vi "ddsRControl.vi"(7 "Pre 3.0 AOM driver version?":bool, 8 "Register":dbl min=0.0 max=16.0 step=1.0 format="%#.1f", 9 "DDS: ProgramChanges":bool, 10 "Lock Amp":bool, 11 "Table/Sequence":bool) -> (0 "Software Trigger":string, 3 "Characters for FPGA":string="L00\r\n")   [LabVIEW 2013, in "DDS9954_v2013.lvlib"]
uses:
  DDS9954_v2013.lvlib
  dataToAscii_8bit.vi
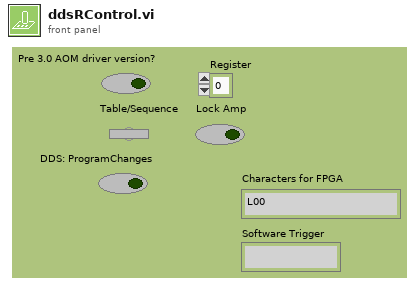
[diagram p1: front panel]
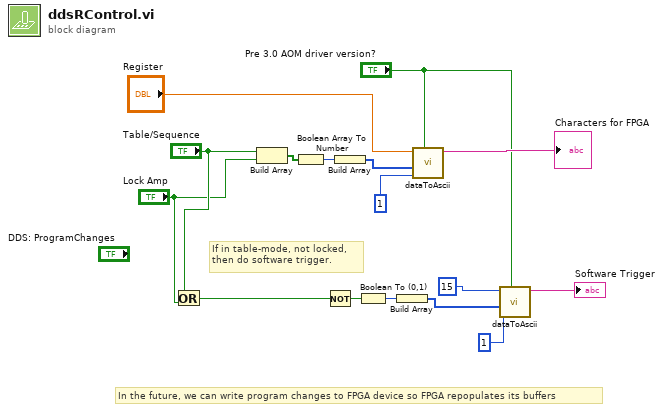
[diagram p0: block diagram]
diagram:
  # "In the future, we can write program changes to FPGA device so FPGA repopulates its buffers"
  # "If in table-mode, not locked,\nthen do software trigger."
  n1 = Or(x="Table/Sequence", y="Lock Amp") -> (x .or. y?=w13:bool)
  n2 = Build Array("Table/Sequence", "Lock Amp") -> (w16:bool[])
  n3 = Boolean Array To Number(Boolean array=w16) -> (number=w11:u32)
  n4 = Not(x=w13) -> (.not. x?=w12:bool)
  n5 = Build Array(w11) -> (w4:u32[])
  n6 = Boolean To (0,1)(Boolean=w12) -> (0, 1=w7:i16)
  n7 = Build Array(w7) -> (w5:i16[])
  n8 = call-poly "dataToAscii.vi"("Pre 3.0 AOM driver version?"="Pre 3.0 AOM driver version?", "HEX min width (pre 3.0)"=u8 1, "Input Data"=w4, "Register"="Register") -> ("Characters to FPGA"=→"Characters for FPGA":string)  [unwired: 7 in]
  n9 = call-poly "dataToAscii.vi"("Pre 3.0 AOM driver version?"="Pre 3.0 AOM driver version?", "HEX min width (pre 3.0)"=u8 1, "Input Data"=w5, "Register"=u8 15 ("unsigned 8bit integer")) -> ("Characters to FPGA"=→"Software Trigger":string)  [unwired: 7 in]
